vi "OCR.vi"(8 "error in (no error)":errorcluster) -> (0 "error out":errorcluster, 3 "Read String":string)   [LabVIEW 2020]
doc: "Reads characters in a region of the image."
uses:
  <vilib>/vision/NI_Vision_Development_Module.lvlib
panel:
  out "Application Directory":path
  out "Image Source":T1(plugin-control)
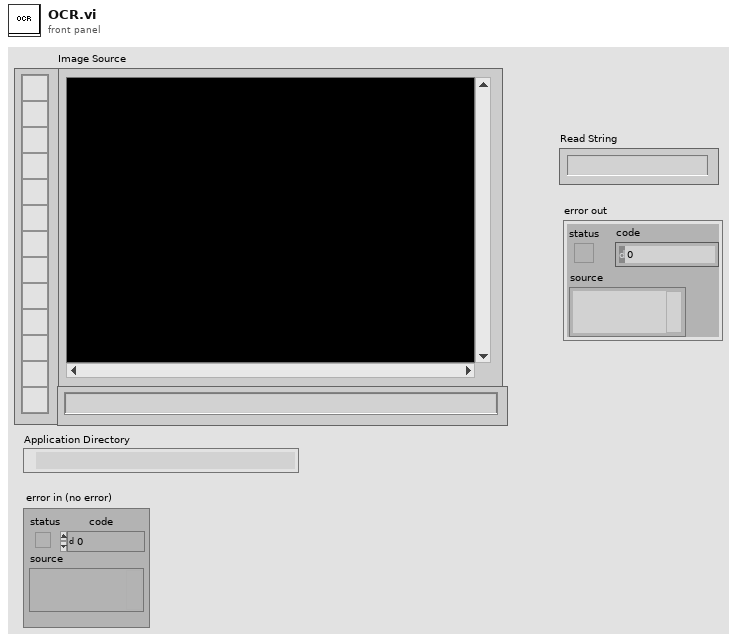
[diagram p1: front panel]
types:
  T1 = typedef "IMAQ Image.ctl" = refnum<image>
  T2 = typedef "IMAQ Rectangle" = cluster{"Left":i32, "Top":i32, "Right":i32, "Bottom":i32, "Rotation":dbl}
  T3 = typedef "IMAQ OCR Session.ctl" = refnum<k1>
  T4 = typedef "ROI Descriptor" = cluster{"Global Rectangle":i32[], "Contours":cluster{"ID":enum32{"External", "Internal"}, "Type":u32, "Coordinates":i32[]}[]}
  T5 = cluster{"Global Rectangle":i32[], "Contours":cluster{"ID":enum32{"External", "Internal"}, "Type":u32, "Coordinates":i32[]}[]}
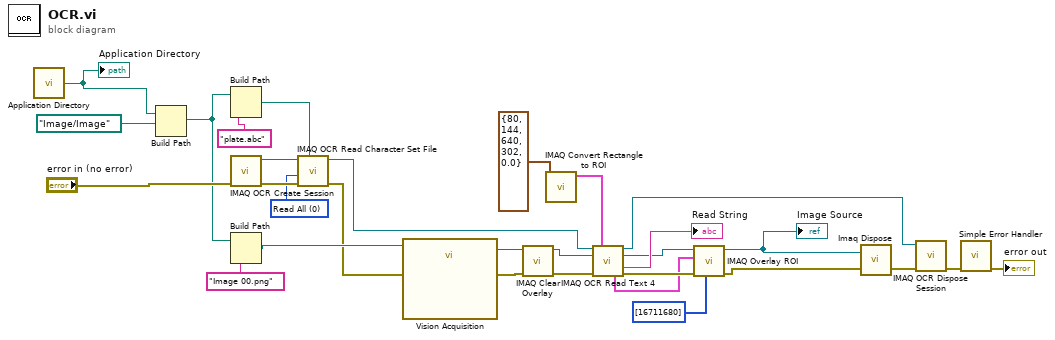
[diagram p0: block diagram]
diagram:
  w27 = 0 items=["Read All", "Read Character Set Only", "Read Properties Only"] ("Read Options")
  n1 = call <vilib>:"Application Directory.vi"() -> ("Application Directory"=w2:path)
  "Application Directory" <- w2
  n2 = Build Path(base path=w2, name or relative path=path "Image/Image") -> (appended path=w4:path)
  n3 = Build Path(base path=w4, name or relative path="plate.abc") -> (appended path=w28:path)
  n4 = call "IMAQ OCR Create Session"("error in (no error)"="error in (no error)") -> ("error out"=w29:errorcluster, "IMAQ OCR Session"=w30:T3)  [unwired: 9 out]
  n5 = Build Path(base path=w4, name or relative path="Image 00.png") -> (appended path=w9:path)
  n6 = call "IMAQ OCR Read Character Set File"("File Path"=w28, "error in (no error)"=w29, "Read Options"=w27, "IMAQ OCR Session"=w30) -> ("error out"=w1:errorcluster, "IMAQ OCR Session (dup)"=w10:T3)  [unwired: 1 in, 5 out]
  n7 = call "Vision Acquisition"("Image Path"=w9, "error in"=w1) -> ("Image Out"=w18:T1, "error out"=w19:errorcluster)  [unwired: 24 in]
  n8 = call "IMAQ Clear Overlay"("error in (no error)"=w19, "Image"=w18) -> ("error out"=w16:errorcluster, "Image Out"=w14:T1)  [unwired: 1 in, 7 out]
  n9 = call "IMAQ Convert Rectangle to ROI"("Rectangle"=T2 {"Left"=80, "Top"=144, "Right"=640, "Bottom"=302, "Rotation"=0.0}) -> ("ROI Descriptor"=w6:T4)  [unwired: 8 in, 1 out]
  n10 = call "IMAQ OCR Read Text 4"("IMAQ OCR Session"=w10, "ROI Descriptor"=w6, "Image"=w14, "error in (no error)"=w16) -> ("IMAQ OCR Session (dup)"=w5:T3, "Image (dup)"=w13:T1, "Read String"=→"Read String":string, "ROI Bounding Characters"=w11:T5, "error out"=w17:errorcluster)  [unwired: 5 in, 2 out]
  n11 = call "IMAQ Overlay ROI"("Colors (Green)"=u32[] [16711680], "error in (no error)"=w17, "ROI Descriptor"=w11, "Image"=w13) -> ("error out"=w7:errorcluster, "Image Out"=w8:T1)  [unwired: 2 in, 4 out]
  "Image Source" <- w8
  n12 = call "Imaq Dispose"("Image"=w8, "error in (no error)"=w7) -> ("error out"=w24:errorcluster)  [unwired: 1 in, 3 out]
  n13 = call "IMAQ OCR Dispose Session"("error in (no error)"=w24, "IMAQ OCR Session"=w5) -> ("error out"=w25:errorcluster)  [unwired: 9 out]
  n14 = call <vilib>:"Simple Error Handler.vi"("error in (no error)"=w25) -> ("error out"=→"error out":errorcluster)  [unwired: 4 in, 4 out]
